vi "Map Relays to Controls.vi"(8 "error in (no error)":errorcluster, 11 "SwitchMatrix in":refnum<class "SwitchMatrix.lvclass">) -> (0 "error out":errorcluster, 3 "SwitchMatrix out":refnum<class "SwitchMatrix.lvclass">)   [LabVIEW 2019, in "SwitchMatrix.lvlib" / "SwitchMatrix.lvclass"]
uses:
  Library/SwitchMatrix.lvclass
  Library/SwitchMatrix.lvclass/SwitchMatrix.ctl
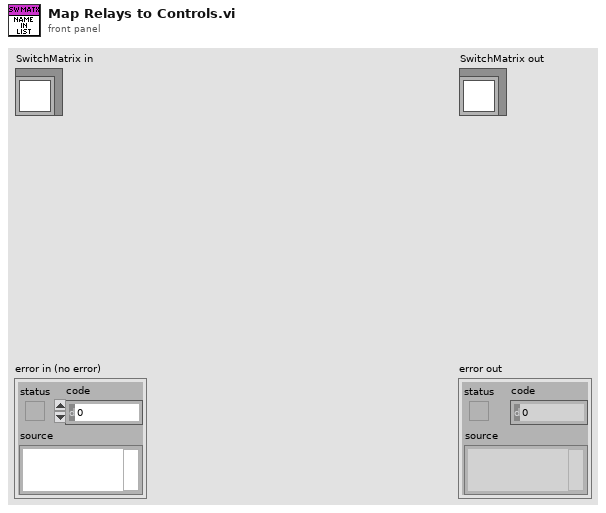
[diagram p1: front panel]
types:
  T1 = typedef "SwitchMatrix.lvlib/SwitchMatrix.lvclass/Topology_Mode.ctl" = enum16{"Single", "Dual", "Quad", "Octal", "Sixteen"}
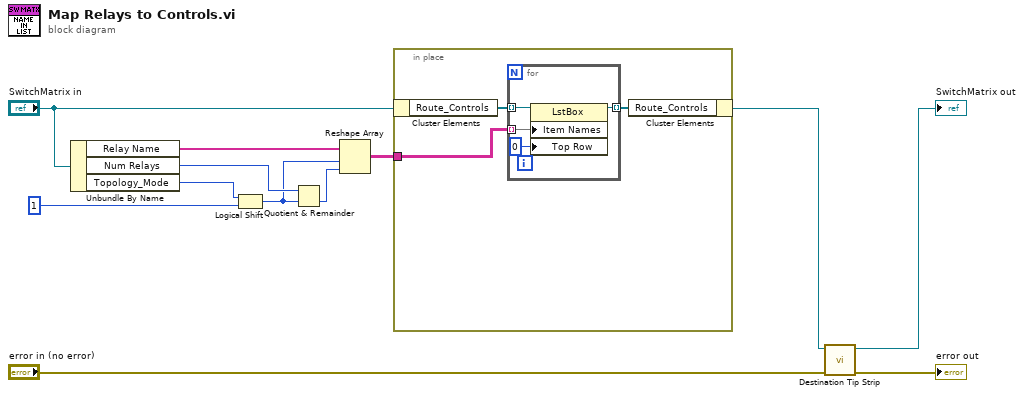
[diagram p0: block diagram]
diagram:
  n1 = Unbundle By Name("SwitchMatrix in") -> ("Relay Name"=w9:string[], "Num Relays"=w10:i32, "Topology_Mode"=w11:T1)
  n2 = Logical Shift(y=w11, x=1) -> (x << y=w8:i32)
  n3 = Quotient & Remainder(x=w10, y=w8) -> (floor(x/y)=w7:i32)  [unwired: 1 out]
  n4 = Reshape Array(w9, w8, w7) -> (w5:string[][])
  n5 = in-place {
    in-place-border: w5 -> [w13]
    n6 = in-place-cluster #1("SwitchMatrix in") -> ("Route_Controls"=w15:refnum<vi>[])
    n7 = for {
      tunnel: w15 -> [w19] mode=indexing
      tunnel: [w18] -> w14 mode=indexing
      tunnel: w13 -> [w17] mode=indexing
      n8 = property class="LstBox"(reference=w19, "Item Names"=w17, "Top Row"=0) -> (reference out=w18:refnum<vi>)  [unwired: 1 in, 1 out]
    }
    n9 = in-place-cluster #1("Route_Controls"=w14) -> (w2:refnum<class "SwitchMatrix.lvclass">)
  }
  n10 = call "Destination Tip Strip.vi"("error in"="error in (no error)", "SwitchMatrix in"=w2) -> ("error out"=→"error out":errorcluster, "SwitchMatrix out"=→"SwitchMatrix out":refnum<class "SwitchMatrix.lvclass">)  [unwired: 8 in]
